vi "Output Multiple Pulses Simple.vi"() -> ()   [LabVIEW 2023]
uses:
  <vilib>/DAQmx/create/channels.llb/DAQmx Create Channel (CO-Pulse Generation-Time).vi
  <vilib>/DAQmx/configure/timing.llb/DAQmx Timing (Implicit).vi
  <resource>/objmgr/daqmx.rc
panel:
  in  "low time":dbl=0.1 format="%.6f"
  in  "high time":dbl=0.1 format="%.6f"
  out "error out":errorcluster
  in  "# of pulses":i32=10
  in  "Pulse Output terminal":tag="/Dev1/PFI3"
  in  "Physical Channel":tag="Dev1/ctr1"
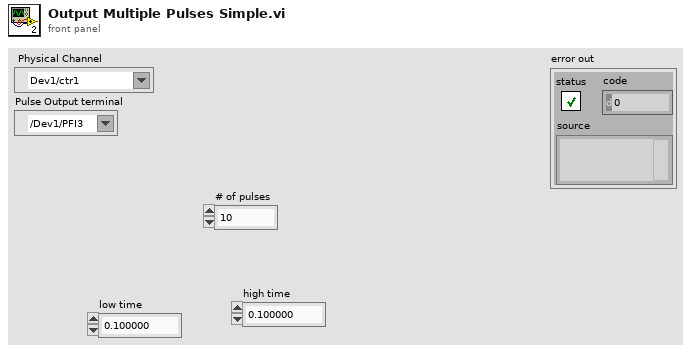
[diagram p1: front panel]
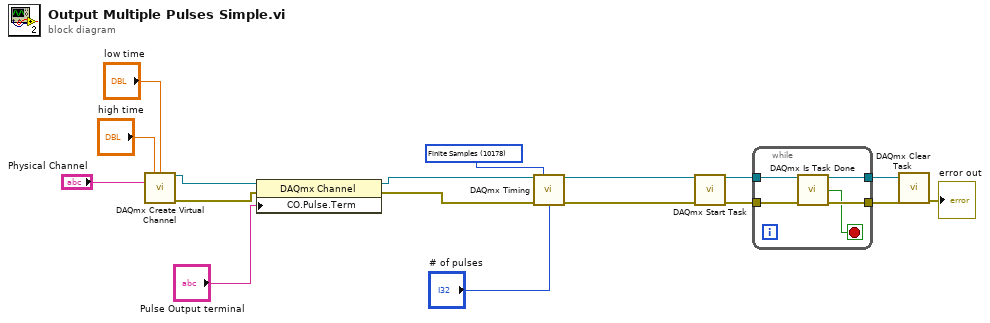
[diagram p0: block diagram]
diagram:
  w15 = 10178 items=["Finite Samples"=10178, "Continuous Samples"=10123, "Hardware Timed Single Point"=12522] ("sample mode")
  n1 = call-poly <vilib>:"DAQmx Create Virtual Channel.vi"("high time"="high time", "low time"="low time", "counter"="Physical Channel") -> ("task out"=w14:refnum<k21>, "error out"=w11:errorcluster)  [unwired: 6 in, 5 out]
  n2 = property class="DAQmx Channel"(reference=w14, error in=w11, "CO.Pulse.Term"="Pulse Output terminal") -> (reference out=w13:refnum<k21>, error out=w12:errorcluster)
  n3 = call-poly <vilib>:"DAQmx Timing.vi"("task/channels in"=w13, "sample mode"=w15, "samples per channel"="# of pulses", "error in"=w12) -> ("task out"=w16:refnum<k21>, "error out"=w8:errorcluster)  [unwired: 4 in, 6 out]
  n4 = call <vilib>:"DAQmx Start Task.vi"("task/channels in"=w16, "error in"=w8) -> ("task out"=w4:refnum<k21>, "error out"=w3:errorcluster)  [unwired: 12 out]
  n5 = while {
    tunnel: w4 -> [w22]
    tunnel: w3 -> [w21]
    tunnel: [w20] -> w2
    tunnel: [w19] -> w1
    stop <- w18 stop-if-true
    n6 = call <vilib>:"DAQmx Is Task Done.vi"("task/channels in"=w22, "error in"=w21) -> ("task out"=w20:refnum<k21>, "task done?"=w18:bool, "error out"=w19:errorcluster)  [unwired: 11 in]
  }
  n7 = call <vilib>:"DAQmx Clear Task.vi"("task in"=w2, "error in"=w1) -> ("error out"=→"error out":errorcluster)  [unwired: 13 out]
